vi "NI6602.constructor.vi"(0 "name":string, 2 "data in":string, 5 "error in (no error)":errorcluster) -> (14 "i ref out":refnum<vi>, 16 "data out":string, 19 "error out":errorcluster)   [LabVIEW 2014, in "NI6602.lvlib"]
doc: "This is the constructor of a class.\n\nLicense Agreement for this software:\n\nCopyright (C)\nGesellschaft für Schwerionenforschung, GSI\nPlanckstr. 1\n64291 Darmstadt\nGermany\n\nContact: D.Beck@gsi.de \n\nThis program is free software; you can redistribute it and/or modify it under the terms of the \nGNU General Public License as published by the Free Software Foundation; either version 2 of \nthe license, or (at your option) any later version.\n\nThis program is distributed in the hope that it will be useful, but WITHOUT ANY WARRANTY; \nwithout even the implied warranty of MERCHANTABILITY or FITNESS FOR A PARTICULAR PURPOSE. See the GNU General License for more details (http://www.gnu.org).\n\nGesellschaft für Schwerionenforschung, GSI\nPlanckstr. 1, 64291 Darmstadt, Germany\nFor all questions and ideas contact: M.Richter@gsi.de, H.Brand@gsi.de or D.Beck@gsi.de.\nLast update: 16-JUN-2004"
uses:
  NI6602.lvlib
  CS_Core/CSApplicationBaseClasses/DeviceBase/DeviceBase.lvlib
  CS_Core/CSSystem/CSSystemLib/CSSystemLib.lvlib
  CS_Core/CSApplicationBaseClasses/DeviceBase/DeviceBase.myEventNames.ctl
  CS_Core/BaseProcess/BaseProcess.lvlib
  CS_Core/CSObj/CSObj.lvlib
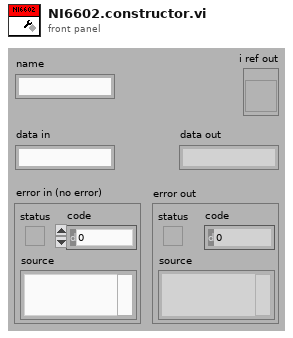
[diagram p1: front panel]
types:
  T1 = enum16{"SetAttribute", "GetAttribute", "CreateAttribute", "DestroyAttribute", "DestroyAllAtributes"}
  T2 = typedef "DeviceBase.lvlib/DeviceBase.myEventNames.ctl" = enum16{"lvmsg://Initialize", "lvmsg://Close", "lvmsg://Configure", "lvmsg://Reset", "lvmsg://IDQuery"}
  T3 = typedef "BaseProcess.lvlib/BaseProcess.i attribute.ctl" = cluster{"EventStatus":string, "EventError":i32, "PresetEvtWatchD":i32, "PresetPdcWatchD":i32, "EventTimeout":i32, "PeriodicInterval":i32, "Interface":string[], "Address":string[], "Special":string[], "PeriodicError":i32, "PeriodicStatus":string, "SuperProc":string, "Descriptors":T4[], "CaseRef":refnum<vi>, "PdcRef":refnum<vi>, "Thread Ref":refnum<vi>, "eventErrorID":i32, "eventStatusID":i32, "periodicErrorID":i32, "periodicStatusID":i32, "pdcCtrID":i32}
  T4 = typedef "BaseProcess.lvlib/BaseProcess.descriptor definition.ctl" = cluster{"selector":string, "descriptor":T5}
  T5 = typedef "BaseProcess.lvlib/BaseProcess.descriptor string definition.ctl" = string
  T6 = typedef "NI6602.lvlib/NI6602.i attribute.ctl" = cluster{"CounterDAQ Channels":cluster{"task":refnum<k21>, "Channel Name":string}[], "RateServiceIDs":i32[], "Running?":bool, "IntegralServiceIDs":i32[], "ThresholdID":i32, "Threshold":dbl, "IntegralValues":dbl[], "Stopped?":bool}
  T7 = typedef "CSObj.lvlib/CSObj.i attribute.ctl" = cluster{"VI Refnum":refnum<vi>, "Front Panel Ref":refnum<vi>, "semaphore":T8, "date of birth":dbl, "ageID":i32, "systemID":i32, "classID":i32, "conditionID":i32, "DefaultPanelType":u16}
  T8 = typedef "Semaphore RefNum" = refnum<k1>
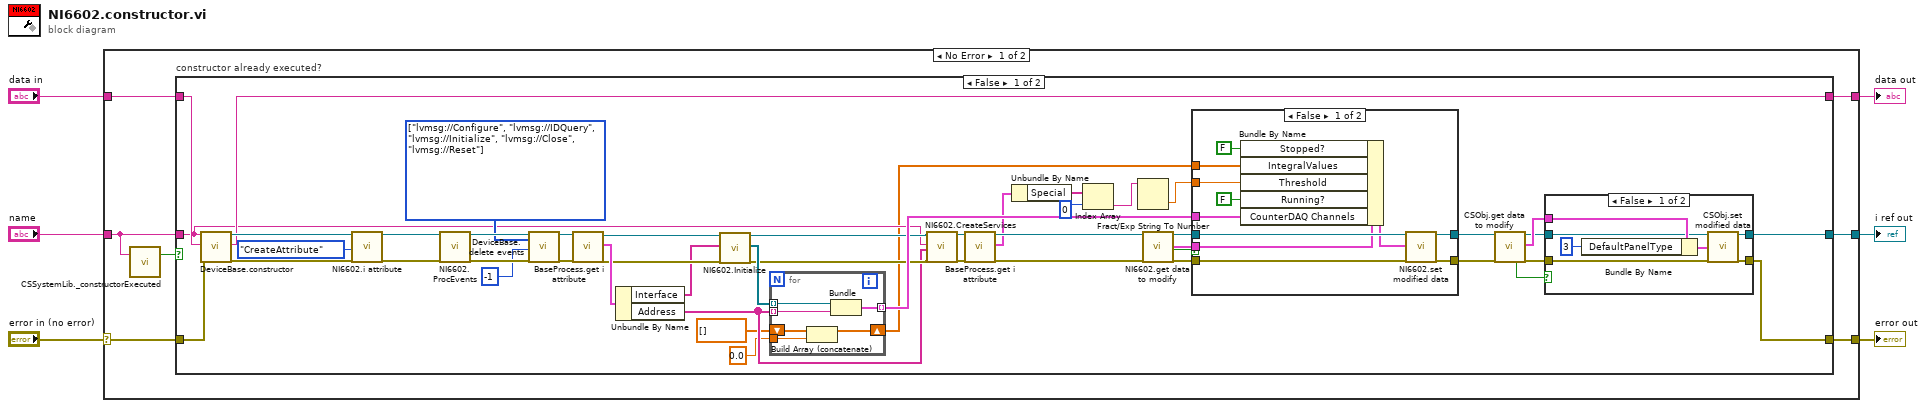
[diagram p0: block diagram]
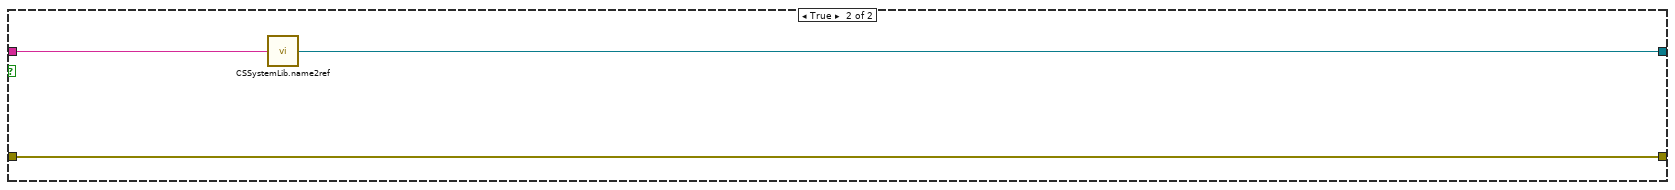
[diagram p4: hidden frame]
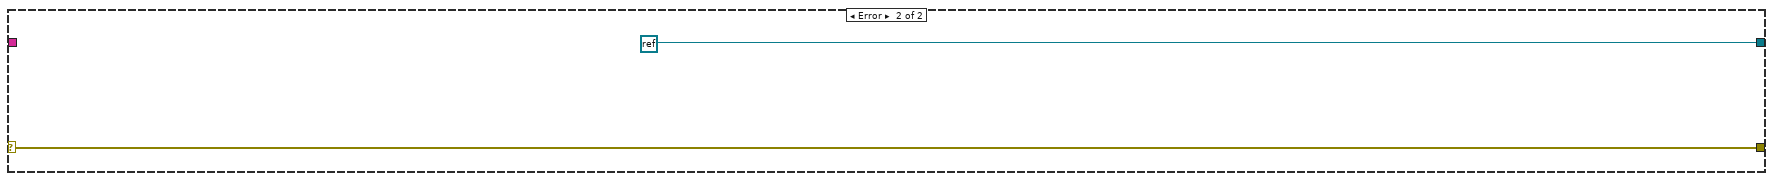
[diagram p5: hidden frame]
diagram:
  n1 = case shown="No Error" "error in (no error)" {
    selector: "error in (no error)" -> [w11 w93]
    tunnel: "name" -> [w10 _]
    tunnel: [w13 refnum<k0> refnum ("Not a Refnum Constant")] -> w5
    tunnel: [w12 w93] -> w4
    tunnel: "data in" -> [w8 _]
    tunnel: [w7 _] -> w1
    frame No Error {
      n2 = call "CSSystemLib._constructorExecuted.vi"("name"=w10) -> ("constructor executed?"=w9:bool)  [unwired: 18 in]
      n3 = case "constructor already executed?" shown="False" w9 {
        tunnel: w10 -> [w35 w92]
        tunnel: [w27 w91] -> w13
        tunnel: [w26 w90] -> w12
        tunnel: w11 -> [w56 w90]
        tunnel: w8 -> [w55 _]
        tunnel: [w50 _] -> w7
        frame False {
          w52 = T2[] [enum."lvmsg://Configure", enum."lvmsg://IDQuery", enum."lvmsg://Initialize", enum."lvmsg://Close", enum."lvmsg://Reset"] items=["lvmsg://Initialize", "lvmsg://Close", "lvmsg://Configure", "lvmsg://Reset", "lvmsg://IDQuery"] ("events")
          n4 = call "DeviceBase.constructor.vi"("name"=w35, "data in"=w55, "error in (no error)"=w56) -> ("i ref out"=w61:refnum<vi>, "data out"=w50:string, "error out"=w60:errorcluster)  [unwired: 14 in]
          n5 = call "NI6602.i attribute.vi"("VI Refnum"=w61, "Action"=T1."CreateAttribute", "error in (no error)"=w60) -> ("VI Refnum out"=w58:refnum<vi>, "error out"=w57:errorcluster)  [unwired: 14 in, 1 out]
          n6 = call "NI6602.ProcEvents.vi"("i ref in"=w58, "error in (no error)"=w57) -> ("i ref out"=w54:refnum<vi>, "error out"=w53:errorcluster)  [unwired: 16 in]
          n7 = call "DeviceBase.delete events.vi"("i ref in"=w54, "events"=w52, "ms timeout (10000)"=-1, "error in (no error)"=w53) -> ("i ref out"=w49:refnum<vi>, "error out"=w48:errorcluster)  [unwired: 13 in, 1 out]
          n8 = call "BaseProcess.get i attribute.vi"("i ref in"=w49, "error in (no error)"=w48) -> ("i ref out"=w42:refnum<vi>, "i attribute"=w47:T3, "error out"=w41:errorcluster)  [unwired: 15 in]
          n9 = Unbundle By Name(w47) -> ("Interface"=w40:string[], "Address"=w34:string[])
          n10 = call "NI6602.Initialize.vi"("i ref in"=w42, "Counter Array"=w40, "error in (no error)"=w41) -> ("i ref out"=w36:refnum<vi>, "Task Array"=w39:refnum<k21>[], "error out"=w37:errorcluster)  [unwired: 14 in]
          n11 = for {
            tunnel: w39 -> [w89] mode=indexing
            tunnel: w34 -> [w88] mode=indexing
            tunnel: [w87] -> w38 mode=indexing
            shift-right: [w85] -> w24
            shift-left: dbl[] [] ("IntegralValues") -> [w86]
            tunnel: 0.0 ("my_serviceID") -> [w84]
            n12 = Build Array (concatenate)(w86, w84) -> (w85:dbl[])
            n13 = Bundle("task out"=w89, "String"=w88) -> (w87:cluster{"task out":refnum<k21>, "String":string})  [unwired: 1 in]
          }
          n14 = call "NI6602.CreateServices.vi"("i ref in"=w36, "name"=w35, "Address"=w34, "error in (no error)"=w37) -> ("i ref out"=w20:refnum<vi>, "error out"=w22:errorcluster)  [unwired: 14 in]
          n15 = call "BaseProcess.get i attribute.vi"("i ref in"=w20, "error in (no error)"=w22) -> ("i ref out"=w19:refnum<vi>, "i attribute"=w18:T3, "error out"=w21:errorcluster)  [unwired: 15 in]
          n16 = Unbundle By Name(w18) -> ("Special"=w17:string[])
          n17 = Index Array(array=w17, index=0) -> (element=w15:string)
          n18 = Fract/Exp String To Number(string=w15) -> (number=w14:dbl)  [unwired: 3 in, 1 out]
          n19 = call "NI6602.get data to modify.vi"("i ref in"=w19, "error in (no error)"=w21) -> ("i ref out"=w46:refnum<vi>, "i attribute"=w43:T6, "timed out"=w44:bool, "error out"=w45:errorcluster)  [unwired: 14 in]
          n20 = case shown="False" w44 {
            tunnel: w46 -> [w81 w83]
            tunnel: [w80 w83] -> w28
            tunnel: w45 -> [w79 w82]
            tunnel: [w78 w82] -> w29
            tunnel: w43 -> [w77 _]
            tunnel: w38 -> [w75 _]
            tunnel: w24 -> [w73 _]
            tunnel: w14 -> [w71 _]
            frame False {
              n21 = Bundle By Name(cluster=w77, "Stopped?"=FALSE, "IntegralValues"=w73, "Threshold"=w71, "Running?"=FALSE, "CounterDAQ Channels"=w75) -> (w76:T6)
              n22 = call "NI6602.set modified data.vi"("i ref in"=w81, "i attribute"=w76, "error in (no error)"=w79) -> ("i ref out"=w80:refnum<vi>, "error out"=w78:errorcluster)  [unwired: 15 in]
            }
            frame True {
            }
          }
          n23 = call "CSObj.get data to modify.vi"("i ref in"=w28, "error in (no error)"=w29) -> ("i ref out"=w31:refnum<vi>, "i attribute"=w33:T7, "timed out"=w30:bool, "error out"=w32:errorcluster)  [unwired: 14 in]
          n24 = case shown="False" w30 {
            tunnel: [w66 w70] -> w27
            tunnel: w31 -> [w67 w70]
            tunnel: [w64 w69] -> w26
            tunnel: w32 -> [w65 w69]
            tunnel: w33 -> [w68 _]
            frame False {
              n25 = Bundle By Name(cluster=w68, "DefaultPanelType"=u16 3) -> (w63:T7)
              n26 = call "CSObj.set modified data.vi"("i ref in"=w67, "i attribute"=w63, "error in (no error)"=w65) -> ("i ref out"=w66:refnum<vi>, "error out"=w64:errorcluster)  [unwired: 15 in]
            }
            frame True {
            }
          }
        }
        frame True {
          n27 = call "CSSystemLib.name2ref.vi"("name"=w92) -> ("obj refnum"=w91:refnum<vi>)
        }
      }
    }
    frame Error {
    }
  }
  "i ref out" <- w5
  "error out" <- w4
  "data out" <- w1
